vi "relay commands to windows PC.vi"(8 "relay data":variant, 9 "relay message":string, 11 "RT Queues":T1) -> (3 "RT Queues out":T1)   [LabVIEW 2018]
uses:
  Type Defs/Queues cluster.ctl
  Chris VIs/Message Scheduler/message scheduler.lvclass
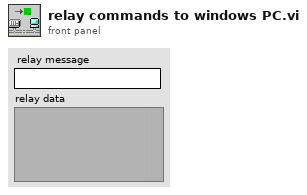
[diagram p1: front panel]
types:
  T1 = typedef "Queues cluster.ctl" = cluster{"RT Message":refnum<queue>, "RT Comms":refnum<queue>, "RT Data":refnum<queue>, "RT FIFO":refnum<queue>, "message scheduler":refnum<class "message scheduler.lvclass">}
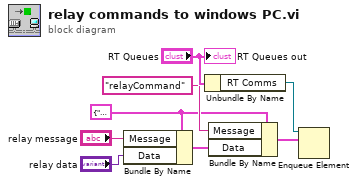
[diagram p0: block diagram]
diagram:
  w4 = cluster{"Message":string, "Data":variant} {"Message"="", "Data"=variant} ("element")
  n1 = Bundle By Name(cluster=w4, "Message"="relay message", "Data"="relay data") -> (w1:cluster{"Message":string, "Data":variant})
  n2 = Unbundle By Name("RT Queues") -> ("RT Comms"=w7:refnum<queue>)
  n3 = Bundle By Name(cluster=w4, "Message"="relayCommand", "Data"=w1) -> (w6:cluster{"Message":string, "Data":variant})
  n4 = Enqueue Element(queue=w7, element=w6) -> ()  [unwired: 2 in, 3 out]
  "RT Queues out" <- "RT Queues"
